vi "Header Data Creator.vi"(0 "tdms file in":refnum<k34>, 1 "Amplifier Metadata":T1 {"Amplifier Model" items=["Select a Model", "AM 1700", "BMA 200"]}, 2 "User Data":T2) -> (7 "tdms file out":refnum<k34>, 10 "error out":errorcluster)   [LabVIEW 2014]
panel:
  # "Outputs"
  # "Blue for On\nOrange for Off"
  # "DC"
  # "AC"
  # "Blue for AC and Orange for DC"
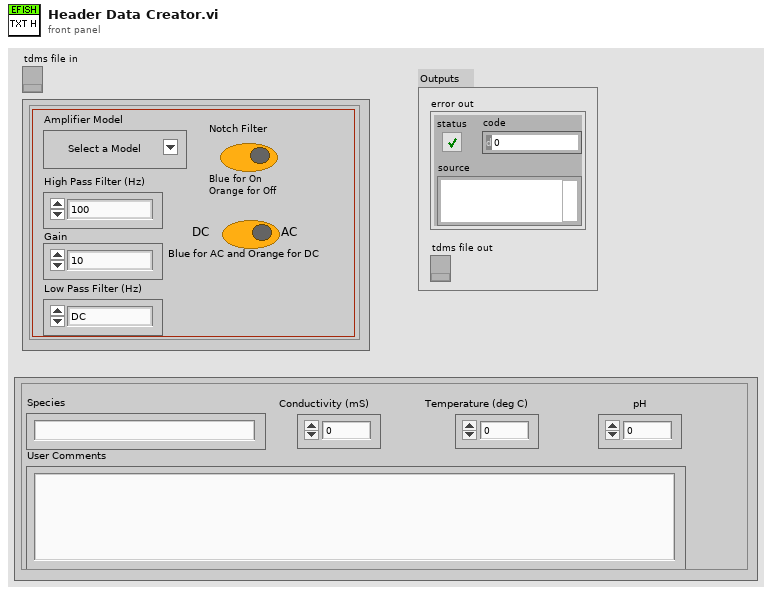
[diagram p1: front panel]
types:
  T1 = cluster{"Low Pass Filter (Hz)":enum16{"DC", "0.1", "1", "3", "10", "30", "100", "300"}, "Gain ":enum16{"10", "20", "50", "100", "200", "500", "1000", "2k", "5k", "10k", "20k", "50k"}, "High Pass Filter (Hz)":enum16{"100", "500", "1000", "3000", "5000", "10,000", "20,000", "30,000", "50,000"}, "Notch Filter":bool, "Amplifier Model":u16, "AC/DC Switch":bool}
  T2 = cluster{"pH":dbl, "Conductivity (mS)":dbl, "Temperature (deg C)":dbl, "User Comments":string, "Species":string}
  T3 = enum16{"DC", "0.1", "1", "3", "10", "30", "100", "300"}
  T4 = enum16{"10", "20", "50", "100", "200", "500", "1000", "2k", "5k", "10k", "20k", "50k"}
  T5 = enum16{"100", "500", "1000", "3000", "5000", "10,000", "20,000", "30,000", "50,000"}
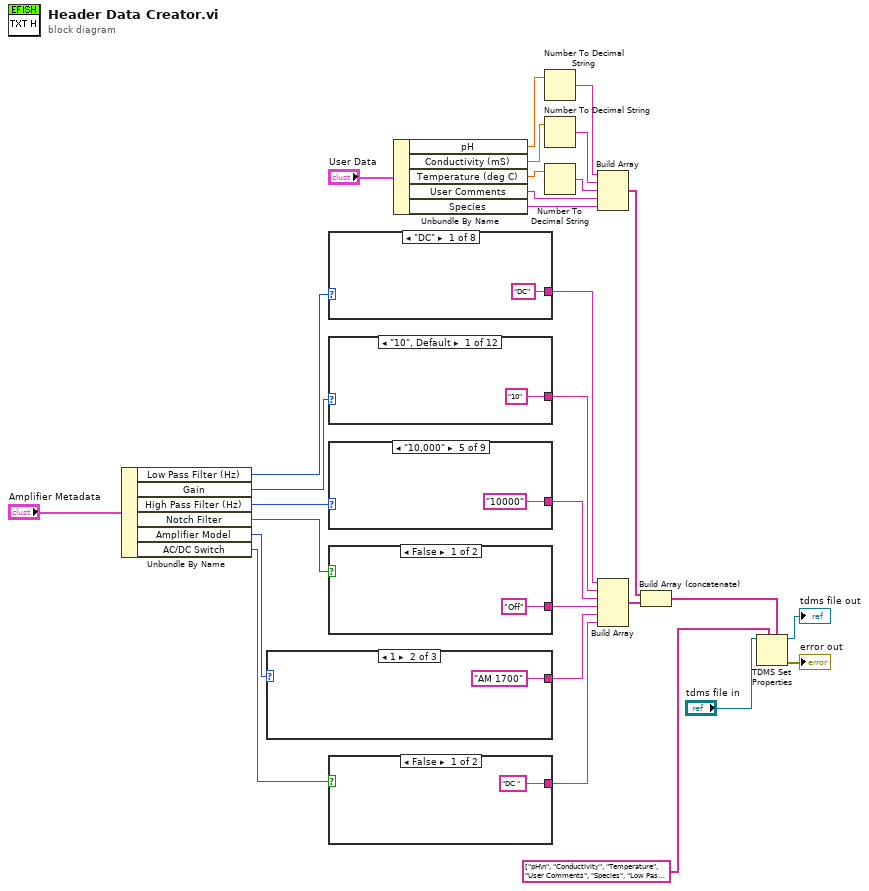
[diagram p0: block diagram]
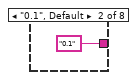
[diagram p2: hidden frame]
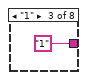
[diagram p3: hidden frame]
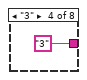
[diagram p4: hidden frame]
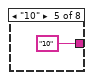
[diagram p5: hidden frame]
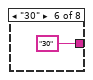
[diagram p6: hidden frame]
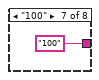
[diagram p7: hidden frame]
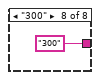
[diagram p8: hidden frame]
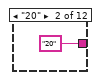
[diagram p9: hidden frame]
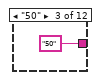
[diagram p10: hidden frame]
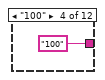
[diagram p11: hidden frame]
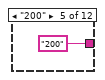
[diagram p12: hidden frame]
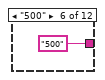
[diagram p13: hidden frame]
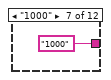
[diagram p14: hidden frame]
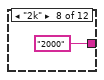
[diagram p15: hidden frame]
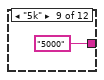
[diagram p16: hidden frame]
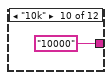
[diagram p17: hidden frame]
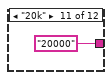
[diagram p18: hidden frame]
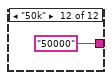
[diagram p19: hidden frame]
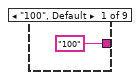
[diagram p20: hidden frame]
diagram:
  n1 = Unbundle By Name("Amplifier Metadata") -> ("Low Pass Filter (Hz)"=w1:T3, "Gain"=w21:T4, "High Pass Filter (Hz)"=w22:T5, "Notch Filter"=w23:bool, "Amplifier Model"=w24:u16, "AC/DC Switch"=w25:bool)
  n2 = case shown="1" w24 {
    tunnel: ["not Selected" ("string") "AM 1700" ("string") "BMA 200" ("string")] -> w10
    frame 0, Default {
    }
    frame 1 {
    }
    frame 2 {
    }
  }
  n3 = case shown="\"DC\"" w1 {
    tunnel: ["DC" ("string") "0.1" ("string") "1" ("string") "3" ("string") "10" ("string") "30" ("string") "100" ("string") "300" ("string")] -> w14
    frame "DC" {
    }
    frame "0.1", Default {
    }
    frame "1" {
    }
    frame "3" {
    }
    frame "10" {
    }
    frame "30" {
    }
    frame "100" {
    }
    frame "300" {
    }
  }
  n4 = case shown="\"10\", Default" w21 {
    tunnel: ["10" ("string") "20" ("string") "50" ("string") "100" ("string") "200" ("string") "500" ("string") "1000" ("string") "2000" ("string") "5000" ("string") "10000" ("string") "20000" ("string") "50000" ("string")] -> w13
    frame "10", Default {
    }
    frame "20" {
    }
    frame "50" {
    }
    frame "100" {
    }
    frame "200" {
    }
    frame "500" {
    }
    frame "1000" {
    }
    frame "2k" {
    }
    frame "5k" {
    }
    frame "10k" {
    }
    frame "20k" {
    }
    frame "50k" {
    }
  }
  n5 = case shown="\"10,000\"" w22 {
    tunnel: ["100" ("string") "1000" ("string") "3000" ("string") "5000" ("string") "10000" ("string") "20000" ("string") "30000" ("string") "50000" ("string") "500 " ("string")] -> w12
    frame "100", Default {
    }
    frame "1000" {
    }
    frame "3000" {
    }
    frame "5000" {
    }
    frame "10,000" {
    }
    frame "20,000" {
    }
    frame "30,000" {
    }
    frame "50,000" {
    }
    frame "500" {
    }
  }
  n6 = case shown="False" w23 {
    tunnel: ["Off" ("string") "On " ("string")] -> w11
    frame False {
    }
    frame True {
    }
  }
  n7 = case shown="False" w25 {
    tunnel: ["DC " "AC "] -> w9
    frame False {
    }
    frame True {
    }
  }
  n8 = Unbundle By Name("User Data") -> ("pH"=w27:dbl, "Conductivity (mS)"=w26:dbl, "Temperature (deg C)"=w20:dbl, "User Comments"=w19:string, "Species"=w18:string)
  n9 = Number To Decimal String(number=w27) -> (decimal integer string=w17:string)  [unwired: 1 in]
  n10 = Number To Decimal String(number=w26) -> (decimal integer string=w16:string)  [unwired: 1 in]
  n11 = Number To Decimal String(number=w20) -> (decimal integer string=w15:string)  [unwired: 1 in]
  n12 = Build Array(w17, w16, w15, w19, w18) -> (w7:string[])
  n13 = Build Array(w14, w13, w12, w11, w10, w9) -> (w8:string[])
  n14 = Build Array (concatenate)(w7, w8) -> (w6:string[])
  n15 = TDMS Set Properties(5:w6, 7:string[] ["pH\n", "Conductivity", "Temperature", "User Comments", "Species", "Low Pass Filter", "Gain", "High Pass Filter", "Notch Filter", "Amplifier Model", "AC / DC Switch"], 11:"tdms file in") -> (0:→"error out":errorcluster, 3:→"tdms file out":refnum<k34>)  [unwired: 3 in, 2 out]
